vi "Get Default FileGlobal and Clone to Active Sequence.vi"(8 "error in (no error)":errorcluster, 10 "FileGlobal to Clone":string, 11 "QPA Measurement in":refnum<class "QPA Measurement.lvclass">) -> (0 "error out":errorcluster, 3 "QPA Measurement out":refnum<class "QPA Measurement.lvclass">)   [LabVIEW 2016, in "QPA Measurement.lvlib" / "QPA Measurement.lvclass"]
uses:
  QPA Measurement.lvclass
  C:/Projects/STS/Common/Sequence Automation/Plugins/Measurement Interface.lvlibp/Measurement Interface.lvclass
  QPA Measurement.lvclass/QPA Measurement.ctl
  Plugins/Measurement Interface.lvlibp/Private Methods/Active Sequence File/Read Active Sequence File.vi
  Plugins/TestStand API Tools (TSAT).lvlibp/TSAT Utilities/TSAT Utilities.lvlib
  Plugins/TestStand API Tools (TSAT).lvlibp/Sequence Actions/TSAT Sequence Actions.lvlib
  Plugins/TestStand API Tools (TSAT).lvlibp/Sequence File Actions/TSAT Sequence File Actions.lvlib
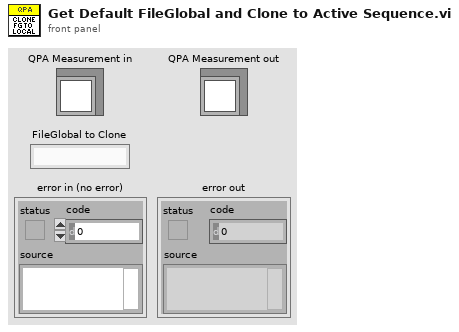
[diagram p1: front panel]
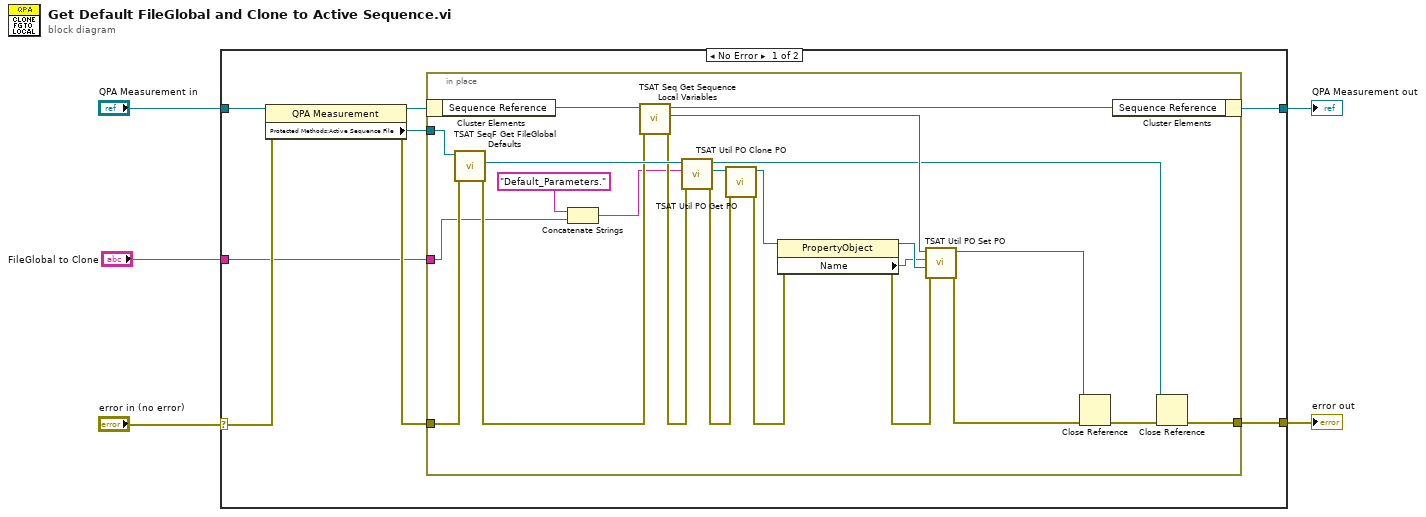
[diagram p0: block diagram]
diagram:
  n1 = case shown="No Error" "error in (no error)" {
    selector: "error in (no error)" -> [w13 w38]
    tunnel: [w8 w38] -> w4
    tunnel: [w6 w37] -> w2
    tunnel: "QPA Measurement in" -> [w12 w37]
    tunnel: "FileGlobal to Clone" -> [w7 _]
    frame No Error {
      n2 = property class="QPA Measurement"(reference=w12, error in=w13) -> (reference out=w11:refnum<class "QPA Measurement.lvclass">, error out=w9:errorcluster, "Protected Methods:Active Sequence File"=w10:refnum<k7>)
      n3 = in-place {
        in-place-border: w10 -> [w32]
        in-place-border: w9 -> [w30]
        in-place-border: [w19] -> w8
        in-place-border: w7 -> [w23]
        n4 = in-place-cluster #1(w11) -> ("Sequence Reference"=w29:refnum<k7>)
        n5 = call "TSAT SeqF Get FileGlobal Defaults.vi"("Error In"=w30, "Sequence File In"=w32) -> ("Error Out"=w28:errorcluster, "FileGlobalsDefaultValues"=w31:refnum<k7>)  [unwired: 7 in, 1 out]
        n6 = Concatenate Strings("Default_Parameters." ("Sub Property to Retrieve"), w23) -> (w24:string)
        n7 = call "TSAT Seq Get Sequence Local Variables.vi"("Error In"=w28, "Sequence Reference In"=w29) -> ("Error Out"=w27:errorcluster, "Locals Out"=w33:refnum<k7>, "Sequence Reference Out"=w22:refnum<k7>)  [unwired: 7 in]
        n8 = call "TSAT Util PO Get PO.vi"("error in (no error)"=w27, "Sub Property to Retrieve"=w24, "Property Object in"=w31) -> ("error out"=w26:errorcluster, "SubProperty"=w35:refnum<k7>, "PropertyObjectOut"=w18:refnum<k7>)  [unwired: 6 in]
        n9 = call "TSAT Util PO Clone PO.vi"("error in (no error)"=w26, "Property Object in"=w35) -> ("error out"=w15:errorcluster, "Clone"=w34:refnum<k7>)  [unwired: 8 in]
        n10 = property class="PropertyObject"(reference=w34, error in=w15) -> (reference out=w17:refnum<k7>, error out=w14:errorcluster, "Name"=w16:string)
        n11 = call "TSAT Util PO Set PO.vi"("error in (no error)"=w14, "newValue"=w17, "Local Variable Name"=w16, "Property Object in"=w33) -> ("error out"=w25:errorcluster, "Property Object Out"=w20:refnum<k7>)  [unwired: 6 in]
        n12 = Close Reference(reference=w20, error in (no error)=w25) -> (error out=w21:errorcluster)
        n13 = in-place-cluster #1("Sequence Reference"=w22) -> (w6:refnum<class "QPA Measurement.lvclass">)
        n14 = Close Reference(reference=w18, error in (no error)=w21) -> (error out=w19:errorcluster)
      }
    }
    frame Error {
    }
  }
  "error out" <- w4
  "QPA Measurement out" <- w2
